vi "Init Enable.vi"(8 "error in (no error)":errorcluster, 11 "[V] Login in":refnum<class "[V] Login.lvclass">) -> (0 "error out":errorcluster, 3 "[V] Login out":refnum<class "[V] Login.lvclass">)   [LabVIEW 2020, in "[V] Login.lvlib" / "[V] Login.lvclass"]
uses:
  [V] Login.lvclass
  [V] Login.lvclass/[V] Login.ctl
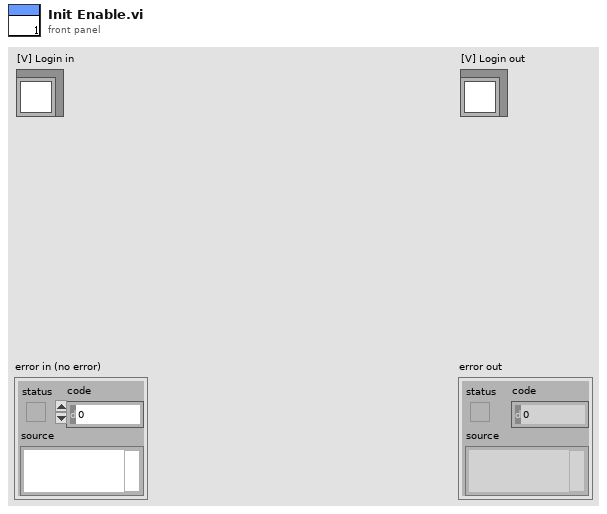
[diagram p1: front panel]
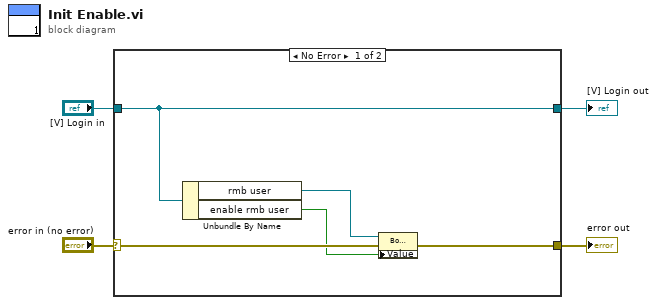
[diagram p0: block diagram]
diagram:
  n1 = case shown="No Error" "error in (no error)" {
    selector: "error in (no error)" -> [w8 w11]
    tunnel: [w5 w11] -> w3
    tunnel: [w9 w10] -> w1
    tunnel: "[V] Login in" -> [w9 w10]
    frame No Error {
      n2 = Unbundle By Name(w9) -> ("rmb user"=w7:refnum<vi>, "enable rmb user"=w6:bool)
      n3 = property class="Bool (strict)"(reference=w7, error in=w8, "Value"=w6) -> (error out=w5:errorcluster)  [unwired: 1 out]
    }
    frame Error {
    }
  }
  "error out" <- w3
  "[V] Login out" <- w1
